vi "F22.vi"(8 "error in":errorcluster, 9 "data":u8[](array[numeric]), 10 "function":u8, 11 "device data model in":refnum<class "Standard Data Model.lvclass">) -> (0 "error out":errorcluster, 1 "data return":u8[](array[numeric]), 2 "function return":u8, 3 "device data model out":refnum<class "Standard Data Model.lvclass">)   [LabVIEW 2012, in "Standard Data Model.lvclass"]
doc: "Executes function code 22"
uses:
  Standard Data Model.lvclass
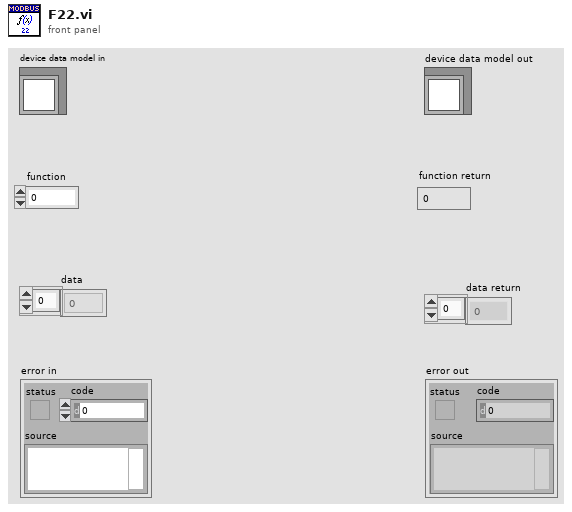
[diagram p1: front panel]
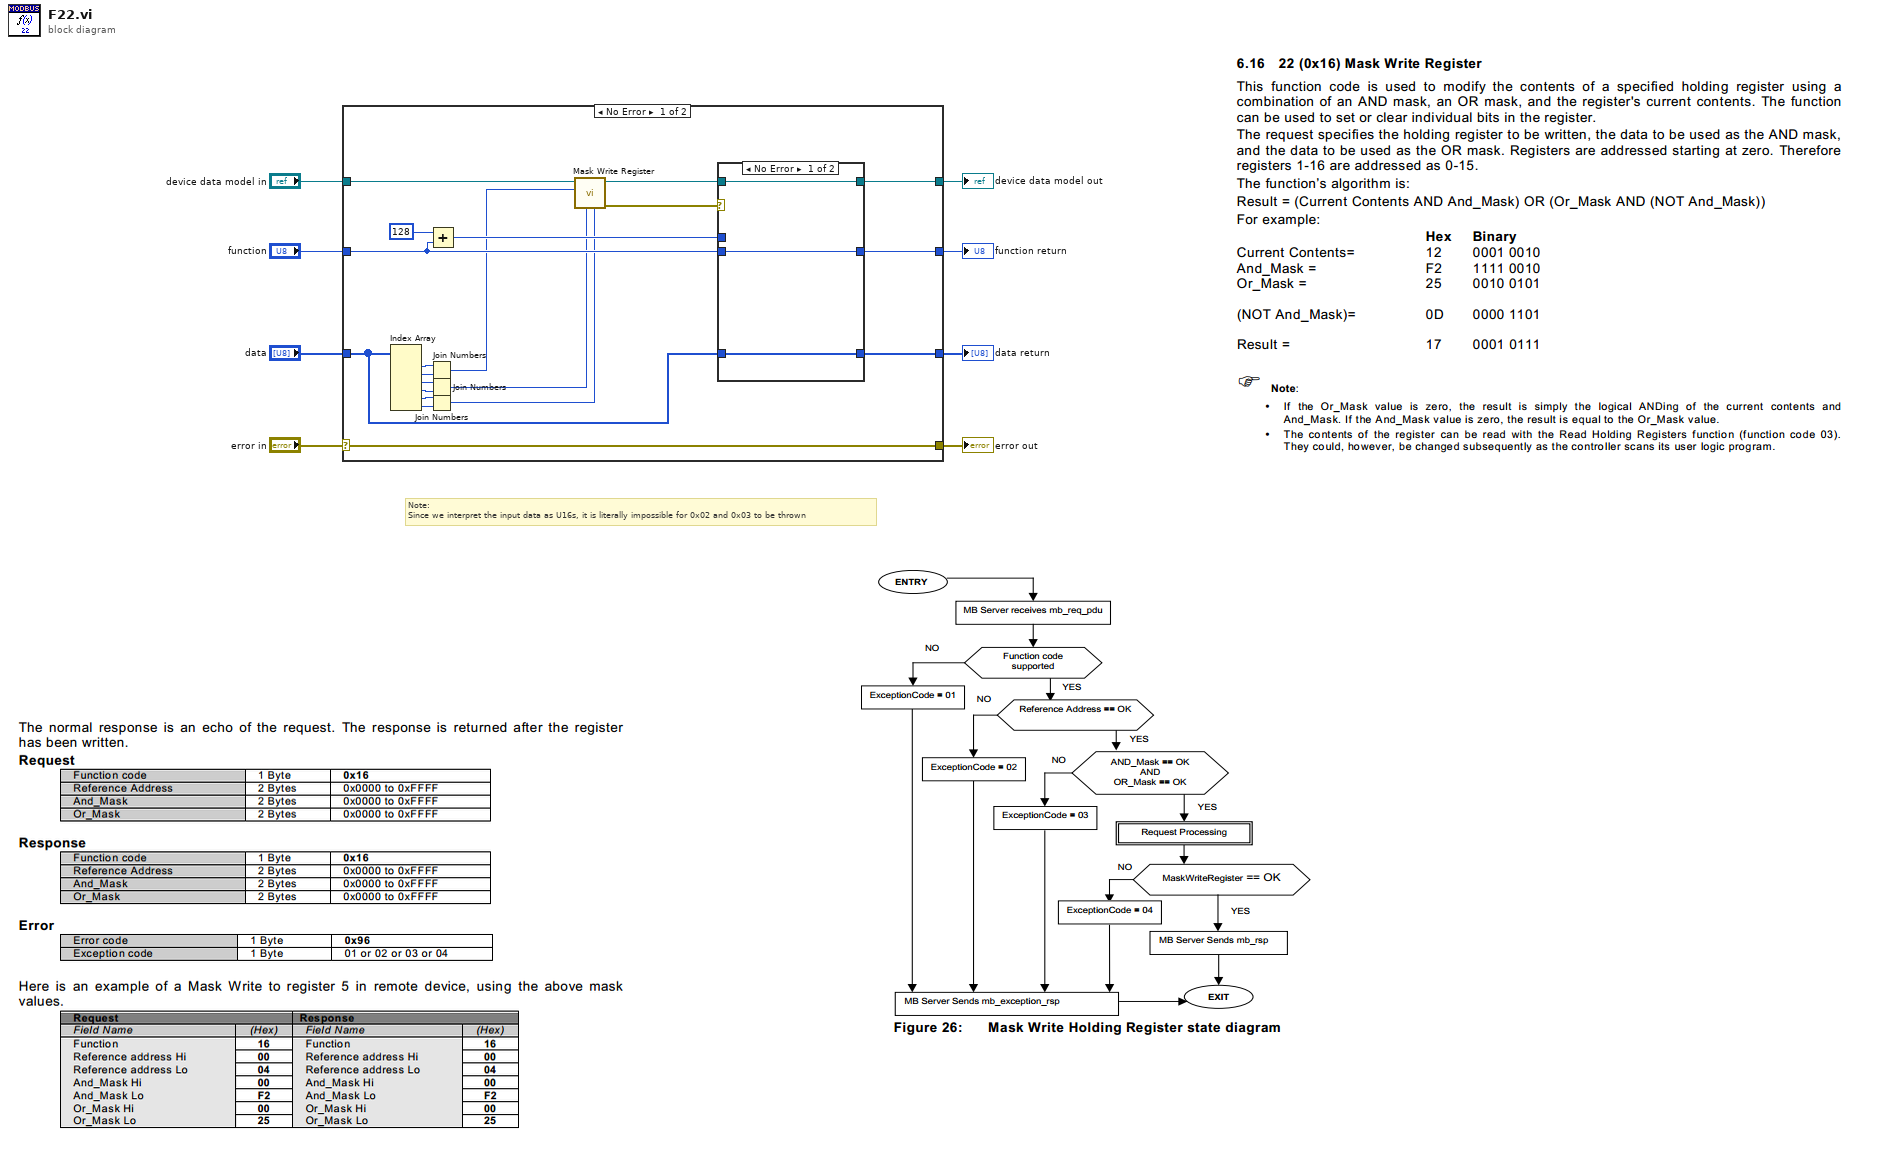
[diagram p0: block diagram]
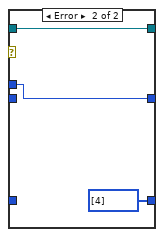
[diagram p2: hidden frame]
diagram:
  # "Note:\nSince we interpret the input data as U16s, it is literally impossible for 0x02 and 0x03 to be thrown"
  n1 = case shown="No Error" "error in" {
    selector: "error in" -> [w28 w38]
    tunnel: [w28 w38] -> w7
    tunnel: [w23 w37] -> w5
    tunnel: "device data model in" -> [w15 w37]
    tunnel: "function" -> [w20 w36]
    tunnel: "data" -> [w9 w35]
    tunnel: [w19 w36] -> w2
    tunnel: [w18 w35] -> w1
    frame No Error {
      n2 = Index Array(array=w9) -> (element #1=w26:u8, element #2=w27:u8, element #3=w25:u8, element #4=w24:u8, element #5=w16:u8, element #6=w17:u8)  [unwired: 6 in]
      n3 = Join Numbers(hi=w26, lo=w27) -> ((hi.lo)=w13:u16)
      n4 = Join Numbers(hi=w25, lo=w24) -> ((hi.lo)=w12:u16)
      n5 = Join Numbers(hi=w16, lo=w17) -> ((hi.lo)=w11:u16)
      n6 = Add(x=u8 128, y=w20) -> (x+y=w21:u8)
      n7 = call-dynamic "Mask Write Register.vi"("OR Mask"=w11, "AND Mask"=w12, "address"=w13, "device data model in"=w15) -> ("error out"=w10:errorcluster, "device data model out"=w14:refnum<class "Standard Data Model.lvclass">)  [unwired: 6 in]
      n8 = case shown="No Error" w10 {
        tunnel: w14 -> [w31 w34]
        tunnel: [w31 w34] -> w23
        tunnel: w21 -> [_ w33]
        tunnel: w20 -> [w30 _]
        tunnel: [w30 w33] -> w19
        tunnel: [w29 u8[] [4]] -> w18
        tunnel: w9 -> [w29 _]
        frame No Error {
        }
        frame Error {
        }
      }
    }
    frame Error {
    }
  }
  "error out" <- w7
  "device data model out" <- w5
  "data return" <- w1
  "function return" <- w2
